vi "driveLoop.vi"() -> ()   [LabVIEW 2018]
uses:
  driveCommandEnum.ctl
  driveShifterEnum.ctl
  <vilib>/Platform/TimedLoop/XDataNode/timing_clust.ctl
  <vilib>/Platform/TimedLoop/XDataNode/nitl_modes.ctl
  <vilib>/Platform/TimedLoop/XDataNode/wakeup.ctl
  <userlib>/836-Library/System/TDMS_V2/Support/TDMS_DevRef.ctl
  <userlib>/836-Library/System/TDMS_V2/Support/Logging_Settings.ctl
  <userlib>/836-Library/System/TDMS_V2/Support/Group_FIFO_Config.ctl
  <userlib>/836-Library/System/TDMS_V2/Support/Channel_FIFO_Config.ctl
  driveStateEnum.ctl
  <vilib>/Rock Robotics/WPI/ThirdParty/Phoenix-LabVIEW/Motor Controller/Controls/CTRE_Phoenix_MotorControl_MotionProfileControlMode.ctl
  Climb/driveClimbStateEnum.ctl
  gear notifier.ctl
  <vilib>/Rock Robotics/WPI/ThirdParty/Phoenix-LabVIEW/Motor Controller/Controls/CTRE_Phoenix_MotorControl_ControlMode.ctl
  <vilib>/Rock Robotics/WPI/ThirdParty/Phoenix-LabVIEW/Motor Controller/Get/CTRE_Phoenix_MotorController_GetVoltage.vi
  <vilib>/addons/control/pid/pid.llb/PID (DBL).vi
  <vilib>/platform/TimedLoop/XDataNode/XDataNode.xnode
  <vilib>/Platform/TimedLoop/XDataNode/XDNodeRunTimeDep.lvlib
  <vilib>/addons/control/pid/NI_PID_pid.lvlib
panel:
  in  "LA limit throt wheel":dbl=0.6
  in  "LA limit throttle":dbl=1.0
  in  "aproachTargetSpeed":dbl=0.64
  in  "sonarBrakeAngleCone":dbl=20.0 format="%#_13g"
  in  "RocketSonarStandOff":dbl=11.0 format="%#_13g"
  in  "coast":dbl=0.08
  in  "alignAngleSetpoint":dbl(slide)=20.0 scale=-30.0..30.0
  in  "Enum":T1
  out "Power output":dbl(graph)=-0.1276953125
  out "Offset Angle":dbl(graph)=4.560546875
  in  "Turn High PID gains":T2={"proportional gain (Kc)"=0.039, "integral time (Ti, min)"=0.0, "derivative time (Td, min)"=0.0018000000000000004} {"derivative time (Td, min)" format="%.4f"; "integral time (Ti, min)" format="%.4f"; "proportional gain (Kc)" format="%.4f"}
  in  "Turn Low PID gains":T2={"proportional gain (Kc)"=0.027999999999999997, "integral time (Ti, min)"=0.0, "derivative time (Td, min)"=0.0018000000000000004} {"derivative time (Td, min)" format="%.4f"; "integral time (Ti, min)" format="%.4f"; "proportional gain (Kc)" format="%.4f"}
  in  "CutoutSonarStandOff":dbl=11.0 format="%#_13g"
  in  "Square?":bool=TRUE
  out "Iteration Duration":i64(graph)=2
  in  "Quickturn_Sens_Low":dbl=1.0
  in  "Quickturn_Sens_High":dbl=0.6 format="%#_13g"
  out "notification":T3=enum."Manuel"
  in  "limit":dbl=1.0
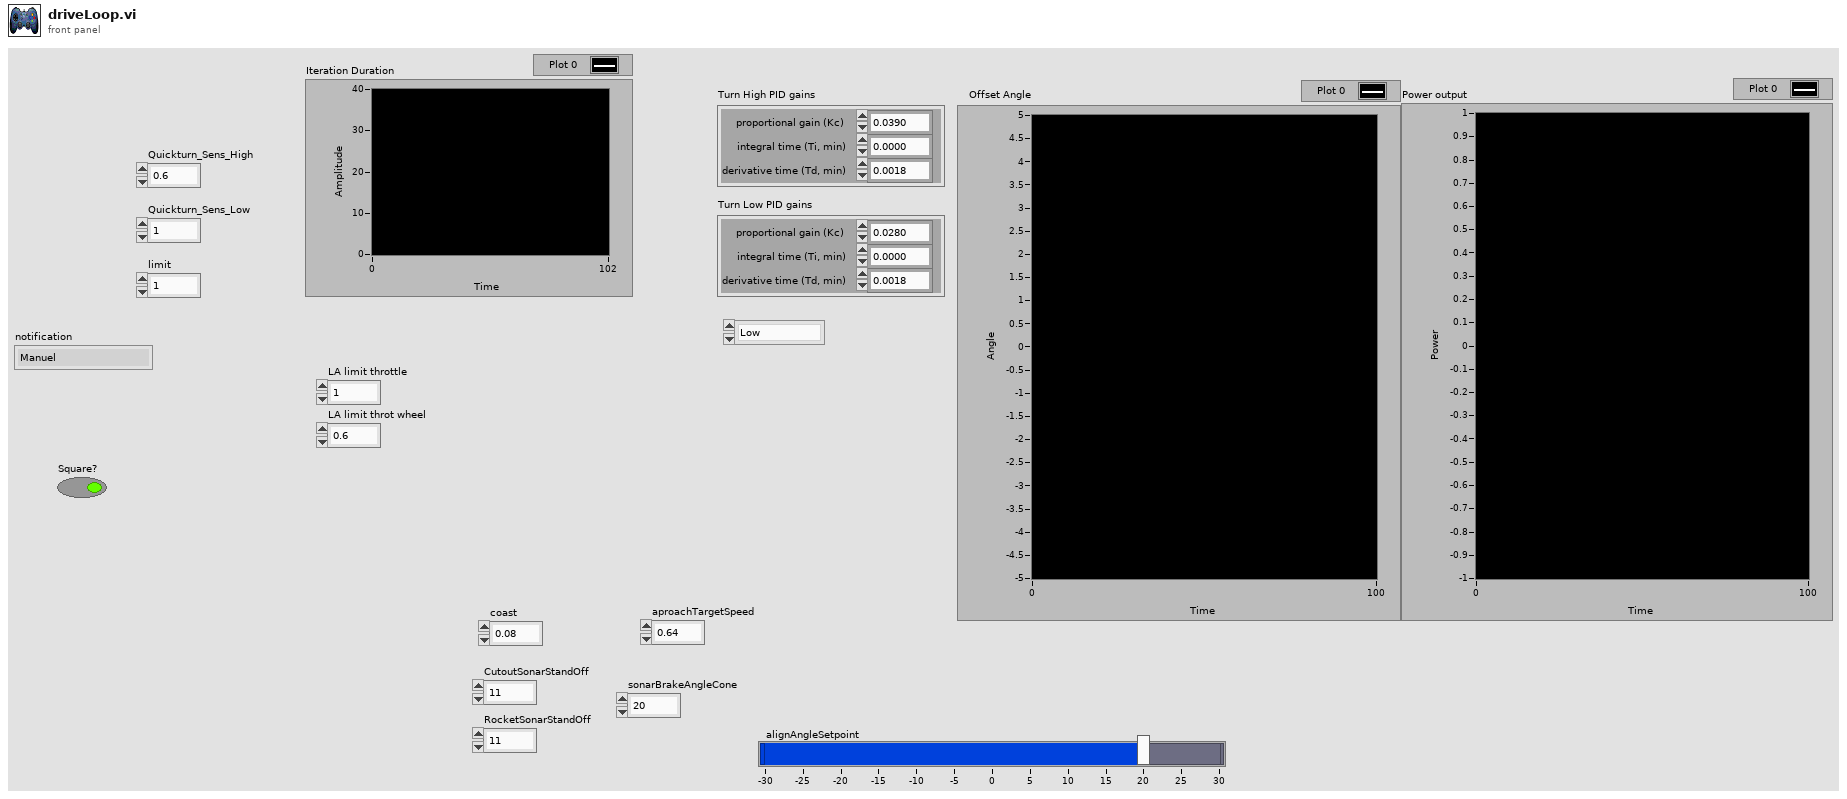
[diagram p1: front panel]
types:
  T1 = typedef "driveShifterEnum.ctl" = enum16{"Low", "High"}
  T2 = cluster{"proportional gain (Kc)":dbl, "integral time (Ti, min)":dbl, "derivative time (Td, min)":dbl}
  T3 = typedef "driveCommandEnum.ctl" = enum16{"doNothing", "Manuel", "Teleop", "Move to Target", "Climb", "Line Align", "Sonar BrakeTele", "Turn To Angle", "Auto Drive", "Test Auto Forward", "Test Auto Reversed", "Code Drive"}
  T4 = typedef "WPI_MotorControlDeviceRef.ctl" = cluster{"DeviceStatus":errorcluster, "Type":T5, "PWM":cluster{"PWM Channel":T6, "DeadBand":T7}, "CAN":cluster{"Device Number":u8, "SetOutput VI Ref":variant, "GetOutput VI Ref":variant, "Enable VI Ref":variant, "Disable VI Ref":variant, "Data":variant}, "Invert":bool, "DIO PWM":cluster{"PWM \"Enable\" Channel":T6, "DIOChannel":T8, "PWM Rate":dbl}}
  T5 = typedef "WPI_MotorControlType.ctl" = enum16{"PWM", "CAN", "DIO PWM"}
  T6 = typedef "FPGA_DIOPWMChannel.ctl" = enum8{"PWM 0", "PWM 1", "PWM 2", "PWM 3", "PWM 4", "PWM 5", "PWM 6", "PWM 7", "PWM 8", "PWM 9", "PWM MXP 0", "PWM MXP 1", "PWM MXP 2", "PWM MXP 3", "PWM MXP 4", "PWM MXP 5", "PWM MXP 6", "PWM MXP 7", "PWM MXP 8", "PWM MXP 9", "Invalid"}
  T7 = typedef "WPI_PWMDeadband.ctl" = cluster{"Name":string, "maxPositivePwm":i32, "minPositivePwm":i32, "centerPwm":i32, "maxNegativePwm":i32, "minNegativePwm":i32, "angularRange":u16}
  T8 = typedef "FPGA_DIOChannel.ctl" = enum8{"DIO 0", "DIO 1", "DIO 2", "DIO 3", "DIO 4", "DIO 5", "DIO 6", "DIO 7", "DIO 8", "DIO 9", "DIO MXP 0", "DIO MXP 1", "DIO MXP 2", "DIO MXP 3", "DIO MXP 4", "DIO MXP 5", "DIO MXP 6", "DIO MXP 7", "DIO MXP 8", "DIO MXP 9", "DIO MXP 10", "DIO MXP 11", "DIO MXP 12", "DIO MXP 13", "DIO MXP 14", "DIO MXP 15", "SPI Port CS1", "SPI Port CS2", "SPI Port CS3", "SPI Port MISO", "SPI Port MOSI", "Invalid"}
  T9 = typedef "CTRE_PigeonIMU_DeviceRef.ctl" = cluster{"DeviceStatus":errorcluster, "Device Number":u8, "Type":T10, "Device ID":u32, "Handle":u64, "UsageFrame":u32, "Library Path":path}
  T10 = typedef "CTRE_PigeonIMU_ConnectionType.ctl" = u32
  T11 = typedef "XDNodeRunTimeDep.lvlib/timing_clust.ctl" = cluster{"Expected End [f-1]":u64, "Actual End [f-1]":u64, "Finished Late? [f-1]":bool, "Expected End [i-1]":u64, "Actual End [i-1]":u64, "Finished Late? [i-1]":bool, "Expected Start [i]":u64, "Actual Start [i]":u64, "Expected Start [f]":u64, "Actual Start [f]":u64, "Source Name":string, "Structure Name":string, "Period":i64, "Deadline":i64, "Offset":i64, "Start":i64, "Priority":i32, "Timeout":i32, "Mode":T12, "Wakeup Reason":T13, "Error":errorcluster, "Source Type":string, "Secondary Source Type":string, "Global End Time":u64, "Global Start Time":u64, "Frame Duration":u64, "Iteration Duration":u64, "Assigned CPU":i32, "I/O Scan Engine Mode":u32}
  T12 = typedef "XDNodeRunTimeDep.lvlib/nitl_modes.ctl" = enum32{"No Change", "Process missed periods, maintain original phase", "Discard missed periods, maintain original phase", "Process missed periods, ignore original phase", "Discard missed periods, ignore original phase"}
  T13 = typedef "XDNodeRunTimeDep.lvlib/wakeup.ctl" = enum32{"Normal", "Aborted", "Asynchronous wakeup", "Timing source error", "Timed loop error", "Timeout"}
  T14 = typedef "driveStateEnum.ctl" = enum16{"doNothing", "Manuel", "Teleop", "Follow Path (init)", "Follow Path", "Move to Target", "Climb", "Line Align", "Turn to Angle", "Sonar Brake Tele", "Code Drive"}
  T15 = enum16{"FollowerType_PercentOutput", "FollowerType_AuxOutput1"}
  T16 = cluster{"Quickturn_Sens_High":dbl, "Quickturn_Sens_Low":dbl}
  T17 = typedef "CTRE_Phoenix_MotorControl_MotionProfileControlMode.ctl" = u16
  T18 = typedef "CTRE_Phoenix_MotorControl_BufferedTrajectoryPointStream_DeviceRef.ctl" = cluster{"Handle":u64, "Library Path":path}
  T19 = typedef "driveClimbStateEnum.ctl" = enum16{"Do Nothing", "Drive Forward"}
  T20 = typedef "gear notifier.ctl" = cluster{"High Gear?":bool, "Low Gear?":bool}
  T21 = typedef "CTRE_Phoenix_MotorControl_ControlMode.ctl" = u16
  T22 = typedef "TDMS_DevRef.ctl" = cluster{"Name":string, "File Ref":refnum<k34>, "Start Time":timestamp, "Logging Settings":T23, "Group FIFO Config":T24[], "Data To Write":refnum<data-value>, "semaphore":T26, "Ref Time Reset":refnum<k4>}
  T23 = typedef "Logging_Settings.ctl" = cluster{"Data Grab Period":dbl, "File Write Period":dbl, "Max Stored Size":dbl, "Burst Size":dbl}
  T24 = typedef "Group_FIFO_Config.ctl" = cluster{"Group":string, "Channels":T25[], "Channel Names":string[]}
  T25 = typedef "Channel_FIFO_Config.ctl" = cluster{"Channel":string, "FIFO":refnum<k33>}
  T26 = typedef "Semaphore RefNum" = refnum<k1>
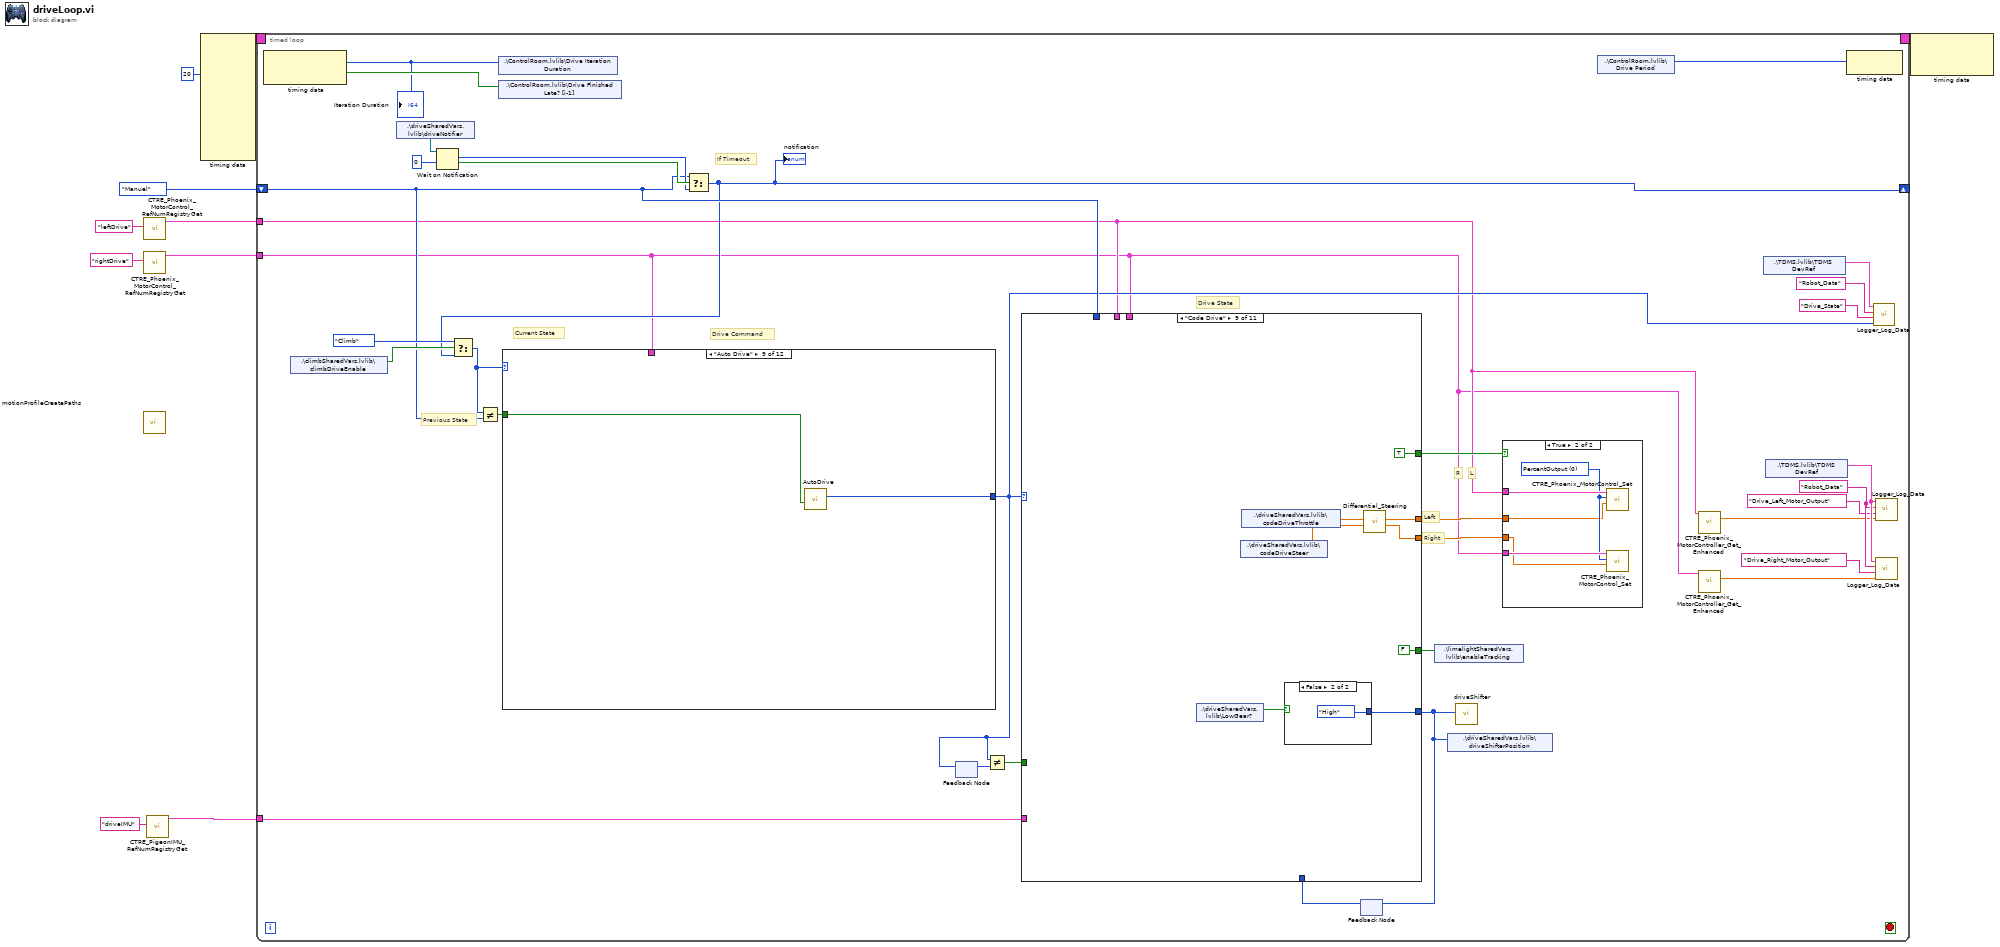
[diagram p0: block diagram]
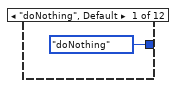
[diagram p2: hidden frame]
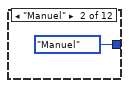
[diagram p3: hidden frame]
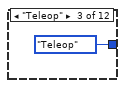
[diagram p4: hidden frame]
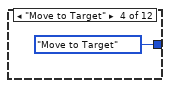
[diagram p5: hidden frame]
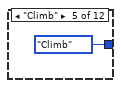
[diagram p6: hidden frame]
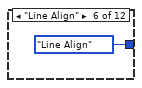
[diagram p7: hidden frame]
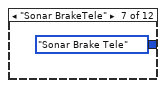
[diagram p8: hidden frame]
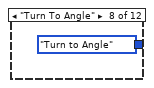
[diagram p9: hidden frame]
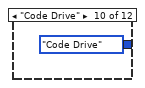
[diagram p10: hidden frame]
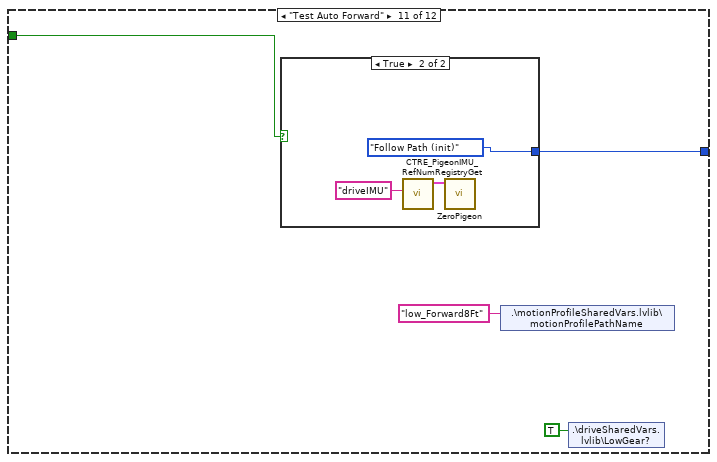
[diagram p11: hidden frame]
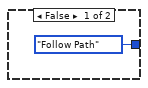
[diagram p12: hidden frame]
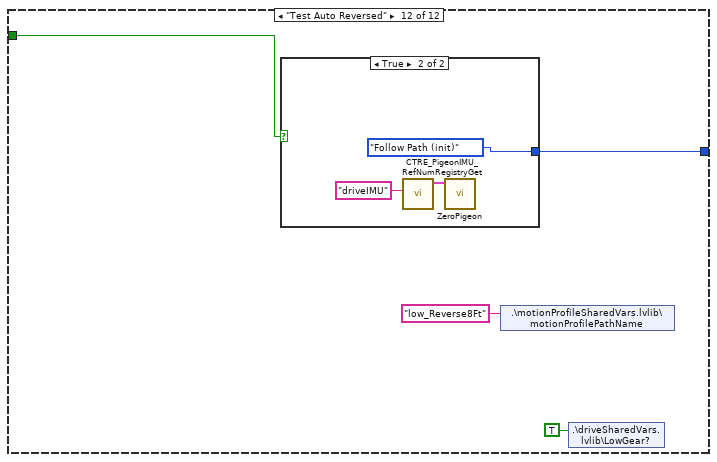
[diagram p13: hidden frame]
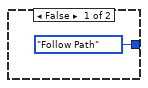
[diagram p14: hidden frame]
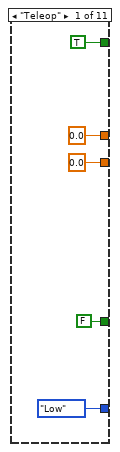
[diagram p16: hidden frame]
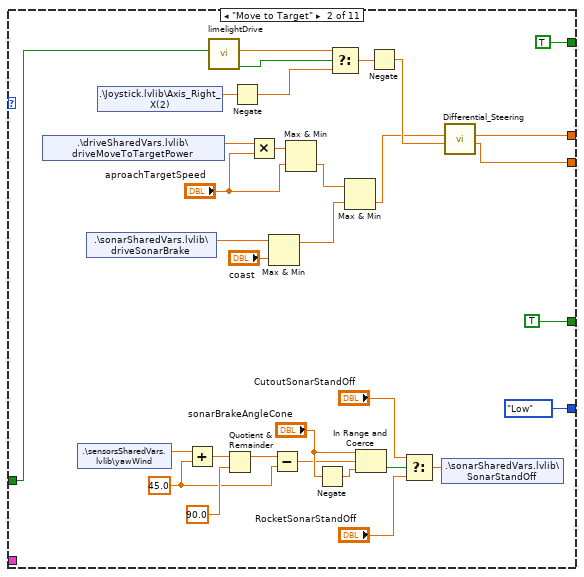
[diagram p17: hidden frame]
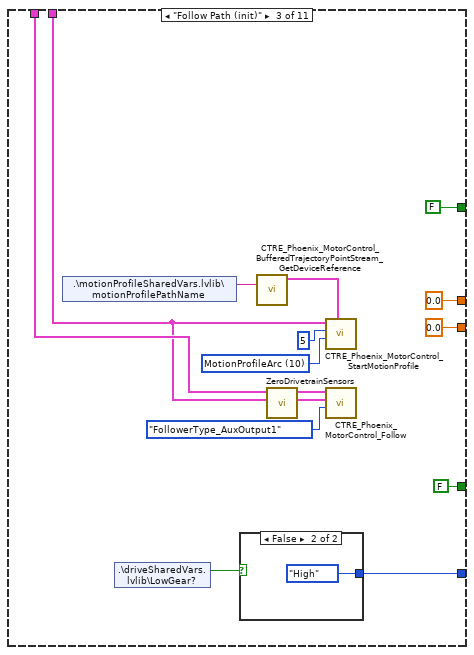
[diagram p18: hidden frame]
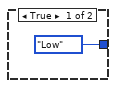
[diagram p19: hidden frame]
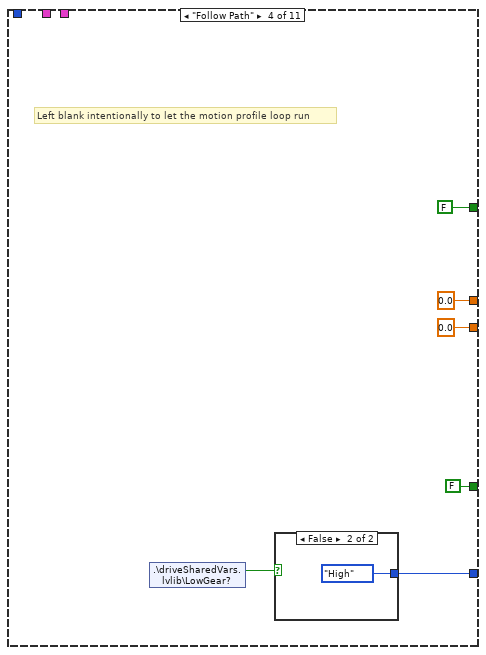
[diagram p20: hidden frame]
diagram:
  n1 = call "motionProfileCreatePaths.vi"() -> ()  [unwired: 12 in]
  n2 = call <vilib>:"CTRE_Phoenix_MotorControl_RefNumRegistryGet.vi"("refnum name"="leftDrive") -> ("PhoenixMotorControlDevRef"=w5:T4)  [unwired: 9 in, 1 out]
  n3 = call <vilib>:"CTRE_Phoenix_MotorControl_RefNumRegistryGet.vi"("refnum name"="rightDrive") -> ("PhoenixMotorControlDevRef"=w4:T4)  [unwired: 9 in, 1 out]
  n4 = call <vilib>:"CTRE_PigeonIMU_RefNumRegistryGet.vi"("refnum name"="driveIMU") -> ("PigeonIMUDevRef"=w2:T9)  [unwired: 9 in, 1 out]
  n5 = node-c288(20 ("Priority")) -> (w10:T11)  [unwired: 9 in]
  n6 = timed-loop {
    timing: w10 -> [_]
    timing-out: [_] -> w9
    shift-right: [w28] -> _
    shift-left: driveCommandEnum."Manuel" ("Drive State Enum") -> [w29]
    tunnel: w5 -> [w12]
    tunnel: w4 -> [w11]
    tunnel: w2 -> [w41]
    stop <- _ stop-if-true
    w22 = "Robot_Data" ("Group")
    # "Drive Command"
    # "Drive State"
    # "Previous State"
    # "Current State"
    # "Right"
    # "Left"
    # "L"
    # "R"
    # "If Timeout"
    n7 = node-c288() -> (w30:i64, w31:bool)  [unwired: 1 in]
    "Iteration Duration" <- w30
    n8 = shared-variable ".\\climbSharedVars.lvlib\\climbDriveEnable"() -> (w36:bool)  [unwired: 1 in, 1 out]
    n9 = shared-variable ".\\driveSharedVars.lvlib\\driveNotifier"() -> (w25:refnum<notifier>)  [unwired: 1 in, 1 out]
    n10 = Wait on Notification(notifier=w25, timeout in ms (-1)=0) -> (notification=w33:T3, timed out?=w44:bool)  [unwired: 2 in, 2 out]
    n11 = shared-variable ".\\ControlRoom.lvlib\\Drive Iteration Duration"(w30) -> ()  [unwired: 1 in, 1 out]
    n12 = shared-variable ".\\ControlRoom.lvlib\\Drive Finished Late? [i-1]"(w31) -> ()  [unwired: 1 in, 1 out]
    n13 = Select(t=w29, s=w44, f=w33) -> (s? t:f=w28:T3)
    "notification" <- w28
    n14 = Select(t=driveCommandEnum."Climb" ("f"), s=w36, f=w28) -> (s? t:f=w38:T3)
    n15 = Not Equal?(x=w38, y=w29) -> (x != y?=w39:bool)
    n16 = case shown="\"Auto Drive\"" w38 {
      tunnel: w39 -> [_ _ _ _ _ _ _ _ w53 _ w59 w67]
      tunnel: [driveStateEnum."doNothing" ("Drive State Enum") driveStateEnum."Manuel" ("Drive State Enum") driveStateEnum."Teleop" ("Drive State Enum") driveStateEnum."Move to Target" ("Drive State Enum") driveStateEnum."Climb" ("Drive State Enum") driveStateEnum."Line Align" ("Drive State Enum") driveStateEnum."Sonar Brake Tele" ("Drive State Enum") driveStateEnum."Turn to Angle" ("Drive State Enum") w54 driveStateEnum."Code Drive" ("Drive State Enum") w58 w66] -> w15
      tunnel: w11 -> [_ _ _ _ _ _ _ _ _ _ _ _]
      frame "doNothing", Default {
      }
      frame "Manuel" {
      }
      frame "Teleop" {
      }
      frame "Move to Target" {
      }
      frame "Climb" {
      }
      frame "Line Align" {
      }
      frame "Sonar BrakeTele" {
      }
      frame "Turn To Angle" {
      }
      frame "Auto Drive" {
        n17 = call "AutoDrive.vi"("Initialized"=w53) -> ("Drive State"=w54:T14)  [unwired: 10 in]
      }
      frame "Code Drive" {
      }
      frame "Test Auto Forward" {
        n18 = case shown="True" w59 {
          tunnel: [driveStateEnum."Follow Path" ("Drive State") driveStateEnum."Follow Path (init)" ("Drive State")] -> w58
          frame False {
          }
          frame True {
            n19 = call <vilib>:"CTRE_PigeonIMU_RefNumRegistryGet.vi"("refnum name"="driveIMU") -> ("PigeonIMUDevRef"=w61:T9)  [unwired: 9 in, 1 out]
            n20 = call "ZeroPigeon.vi"("Pigeon"=w61) -> ()  [unwired: 8 in, 1 out]
          }
        }
        n21 = shared-variable ".\\motionProfileSharedVars.lvlib\\motionProfilePathName"("low_Forward8Ft" ("motionProfilePathName")) -> ()  [unwired: 1 in, 1 out]
        n22 = shared-variable ".\\driveSharedVars.lvlib\\LowGear?"(TRUE ("LowGear?")) -> ()  [unwired: 1 in, 1 out]
      }
      frame "Test Auto Reversed" {
        n23 = case shown="True" w67 {
          tunnel: [driveStateEnum."Follow Path" ("Drive State") driveStateEnum."Follow Path (init)" ("Drive State")] -> w66
          frame False {
          }
          frame True {
            n24 = call <vilib>:"CTRE_PigeonIMU_RefNumRegistryGet.vi"("refnum name"="driveIMU") -> ("PigeonIMUDevRef"=w69:T9)  [unwired: 9 in, 1 out]
            n25 = call "ZeroPigeon.vi"("Pigeon"=w69) -> ()  [unwired: 8 in, 1 out]
          }
        }
        n26 = shared-variable ".\\motionProfileSharedVars.lvlib\\motionProfilePathName"("low_Reverse8Ft" ("motionProfilePathName")) -> ()  [unwired: 1 in, 1 out]
        n27 = shared-variable ".\\driveSharedVars.lvlib\\LowGear?"(TRUE ("LowGear?")) -> ()  [unwired: 1 in, 1 out]
      }
    }
    n28 = feedback-in #1(w15) -> ()
    n29 = feedback #1() -> (w17:T14)  [unwired: 1 in]
    n30 = Not Equal?(x=w15, y=w17) -> (x != y?=w16:bool)
    n31 = feedback #2() -> (w34:T1)  [unwired: 1 in]
    n32 = case shown="\"Code Drive\"" w15 {
      tunnel: [0.0 ("Throttle") w103 0.0 ("Throttle") 0.0 ("Throttle") w141 w156 0.0 ("Throttle") w198 w209 w218 w228] -> w43
      tunnel: [0.0 ("Wheel") w102 0.0 ("Wheel") 0.0 ("Wheel") w141 w155 0.0 ("Wheel") w197 w210 w219 w227] -> w42
      tunnel: w41 -> [_ _ _ _ _ _ _ _ _ _ _]
      tunnel: w12 -> [_ _ w126 _ _ _ _ _ _ _ _]
      tunnel: w11 -> [_ _ w125 _ _ _ _ _ _ _ _]
      tunnel: w29 -> [_ _ _ _ _ _ _ _ _ _ _]
      tunnel: [TRUE ("x .and. y?") TRUE ("x .and. y?") FALSE ("x .and. y?") FALSE ("x .and. y?") TRUE ("x .and. y?") TRUE ("x .and. y?") TRUE ("x .and. y?") TRUE ("x .and. y?") TRUE ("x .and. y?") TRUE ("x .and. y?") TRUE ("x .and. y?")] -> w40
      tunnel: [driveShifterEnum."Low" driveShifterEnum."Low" w114 w131 w143 driveShifterEnum."High" driveShifterEnum."High" w191 w206 driveShifterEnum."Low" ("Enum") "Enum"] -> w35
      tunnel: w34 -> [_ _ _ _ w143 _ _ _ _ _ _]
      tunnel: [FALSE TRUE FALSE FALSE FALSE FALSE FALSE FALSE FALSE FALSE FALSE] -> w27
      tunnel: w16 -> [_ w82 _ _ _ _ _ _ _ w215 _]
      frame "Teleop" {
      }
      frame "Move to Target" {
        w87 = 45.0 ("y")
        n33 = shared-variable ".\\driveSharedVars.lvlib\\driveMoveToTargetPower"() -> (w86:dbl)  [unwired: 1 in, 1 out]
        n34 = shared-variable ".\\sensorsSharedVars.lvlib\\yawWind"() -> (w98:dbl)  [unwired: 1 in, 1 out]
        n35 = shared-variable ".\\sonarSharedVars.lvlib\\driveSonarBrake"() -> (w101:dbl)  [unwired: 1 in, 1 out]
        n36 = shared-variable ".\\Joystick.lvlib\\Axis_Right_X(2)"() -> (w109:dbl)  [unwired: 1 in, 1 out]
        n37 = Add(x=w98, y=w87) -> (x+y=w89:dbl)
        n38 = call "limelightDrive.vi"("reinitialize? (F)"=w82) -> ("Valid Track"=w110:bool, "Turn Output"=w111:dbl)  [unwired: 9 in]
        n39 = Quotient & Remainder(x=w89, y=90.0) -> (x-y*floor(x/y)=w96:dbl)  [unwired: 1 out]
        n40 = Negate(x=w109) -> (-x=w108:dbl)
        n41 = Multiply(x=w86, y="aproachTargetSpeed") -> (x*y=w85:dbl)
        n42 = Max & Min(x=w101, y="coast") -> (max(x,y)=w99:dbl)  [unwired: 1 out]
        n43 = Subtract(x=w96, y=w87) -> (x-y=w88:dbl)
        n44 = Max & Min(x=w85, y="aproachTargetSpeed") -> (min(x,y)=w83:dbl)  [unwired: 1 out]
        n45 = Negate(x="sonarBrakeAngleCone") -> (-x=w94:dbl)
        n46 = Select(t=w111, s=w110, f=w108) -> (s? t:f=w106:dbl)
        n47 = Max & Min(x=w83, y=w99) -> (min(x,y)=w104:dbl)  [unwired: 1 out]
        n48 = In Range and Coerce(upper limit="sonarBrakeAngleCone", x=w88, lower limit=w94) -> (In Range?=w93:bool)  [unwired: 1 out]
        n49 = Negate(x=w106) -> (-x=w105:dbl)
        n50 = Select(t="CutoutSonarStandOff", s=w93, f="RocketSonarStandOff") -> (s? t:f=w92:dbl)
        n51 = shared-variable ".\\sonarSharedVars.lvlib\\SonarStandOff"(w92) -> ()  [unwired: 1 in, 1 out]
        n52 = call <userlib>:"Differential_Steering.vi"("Steer"=w105, "Base"=w104) -> ("Right"=w102:dbl, "Left"=w103:dbl)  [unwired: 4 in]
      }
      frame "Follow Path (init)" {
        w121 = T17 10 items=["MotionProfile"=6, "MotionProfileArc"=10] ("Control Mode")
        n53 = shared-variable ".\\motionProfileSharedVars.lvlib\\motionProfilePathName"() -> (w117:string)  [unwired: 1 in, 1 out]
        n54 = shared-variable ".\\driveSharedVars.lvlib\\LowGear?"() -> (w115:bool)  [unwired: 1 in, 1 out]
        n55 = case shown="False" w115 {
          tunnel: [driveShifterEnum."Low" ("Enum") driveShifterEnum."High" ("Enum")] -> w114
          frame True {
          }
          frame False {
          }
        }
        n56 = call <vilib>:"CTRE_Phoenix_MotorControl_BufferedTrajectoryPointStream_GetDeviceReference.vi"("refnum name"=w117) -> ("BufferedTrajectoryPointStream_DevRef"=w118:T18)  [unwired: 9 in, 1 out]
        n57 = call "ZeroDrivetrainSensors.vi"("Talon 2"=w125, "Talon 1"=w126) -> ("Talon 2"=w119:T4, "Talon 1"=w120:T4)  [unwired: 8 in]
        n58 = call <vilib>:"CTRE_Phoenix_MotorControl_StartMotionProfile.vi"("BufferedTrajectoryPointStream_DevRef"=w118, "Control Mode"=w121, "minBufferedPts"=u32 5, "PhoenixMotorControlDevRef"=w125) -> ()  [unwired: 6 in, 2 out]
        n59 = call <vilib>:"CTRE_Phoenix_MotorControl_Follow.vi"("FollowerType"=T15."FollowerType_AuxOutput1", "Master Controller to Follow"=w119, "PhoenixMotorControlDevRef"=w120) -> ()  [unwired: 7 in, 2 out]
      }
      frame "Follow Path" {
        # "Left blank intentionally to let the motion profile loop run"
        n60 = shared-variable ".\\driveSharedVars.lvlib\\LowGear?"() -> (w132:bool)  [unwired: 1 in, 1 out]
        n61 = case shown="False" w132 {
          tunnel: [driveShifterEnum."Low" ("Enum") driveShifterEnum."High" ("Enum")] -> w131
          frame True {
          }
          frame False {
          }
        }
      }
      frame "Sonar Brake Tele" {
        # "Share Control Authority between\nDriver input and Sonar PID"
        n62 = shared-variable ".\\Joystick.lvlib\\Axis_Left_Y(1)"() -> (w140:dbl)  [unwired: 1 in, 1 out]
        n63 = shared-variable ".\\sonarSharedVars.lvlib\\driveSonarBrake"() -> (w142:dbl)  [unwired: 1 in, 1 out]
        n64 = Negate(x=w140) -> (-x=w139:dbl)
        n65 = Max & Min(x=w139, y=w142) -> (min(x,y)=w141:dbl)  [unwired: 1 out]
      }
      frame "Climb" {
        n66 = shared-variable ".\\driveSharedVars.lvlib\\driveClimbStateNotifier"() -> (w152:refnum<notifier>)  [unwired: 1 in, 1 out]
        n67 = Wait on Notification(notifier=w152, timeout in ms (-1)=0) -> (notification=w148:T19, timed out?=w150:bool)  [unwired: 2 in, 2 out]
        n68 = feedback-in #3(w148) -> ()
        n69 = feedback #3() -> (w147:T19)  [unwired: 1 in]
        n70 = Select(t=w147, s=w150, f=w148) -> (s? t:f=w149:T19)
        n71 = case shown="\"Drive Forward\"" w149 {
          tunnel: [w157 w159] -> w156
          tunnel: [w157 w158] -> w155
          frame "Drive Forward" {
            n72 = shared-variable ".\\climbSharedVars.lvlib\\Drive Speed"() -> (w157:dbl)  [unwired: 1 in, 1 out]
          }
          frame "Do Nothing", Default {
            w158 = 0.0  # Right
            w159 = 0.0  # Left
          }
        }
      }
      frame "doNothing", Default {
      }
      frame "Manuel" {
        n73 = shared-variable ".\\driveSharedVars.lvlib\\driveShifterNotifier"() -> (w165:refnum<notifier>)  [unwired: 1 in, 1 out]
        n74 = shared-variable ".\\Joystick.lvlib\\Axis_Right_X(2)"() -> (w168:dbl)  [unwired: 1 in, 1 out]
        n75 = shared-variable ".\\Joystick.lvlib\\Axis_Left_Y(1)"() -> (w172:dbl)  [unwired: 1 in, 1 out]
        n76 = Wait on Notification(notifier=w165, timeout in ms (-1)=0) -> (notification=w180:T20, timed out?=w179:bool)  [unwired: 2 in, 2 out]
        n77 = Sign(1:w172) -> (0:w176:dbl)
        n78 = Sign(1:w168) -> (0:w174:dbl)
        n79 = Square(x=w172) -> (x^2=w177:dbl)
        n80 = Square(x=w168) -> (x^2=w175:dbl)
        n81 = feedback #4() -> (w178:T20)  [unwired: 1 in]
        n82 = Select(t=w178, s=w179, f=w180) -> (s? t:f=w182:T20)
        n83 = feedback-in #4(w182) -> ()
        n84 = Bundle By Name(cluster=T16 {"Quickturn_Sens_High"=1.0, "Quickturn_Sens_Low"=1.0} ("Sens Values"), "Quickturn_Sens_High"="Quickturn_Sens_High", "Quickturn_Sens_Low"="Quickturn_Sens_Low") -> (w194:T16)
        n85 = Multiply(x=w177, y=w176) -> (x*y=w173:dbl)
        n86 = Multiply(x=w175, y=w174) -> (x*y=w170:dbl)
        n87 = Select(t=w173, s="Square?", f=w172) -> (s? t:f=w171:dbl)
        n88 = Select(t=w170, s="Square?", f=w168) -> (s? t:f=w169:dbl)
        n89 = Unbundle By Name(w182) -> ("High Gear?"=w183:bool, "Low Gear?"=w184:bool)
        n90 = Negate(x=w171) -> (-x=w202:dbl)
        n91 = Multiply(x=w202, y="limit") -> (x*y=w166:dbl)
        n92 = Multiply(x="limit", y=w169) -> (x*y=w199:dbl)
        n93 = call <userlib>:"JK_Latch.vi"("Reset"=w183, "Set"=w184) -> ("Q"=w185:bool)  [unwired: 5 in]
        n94 = Select(t=driveShifterEnum."Low", s=w185, f=driveShifterEnum."High") -> (s? t:f=w191:T1)
        n95 = case shown="\"Low\"" w191 {
          tunnel: [enum16{"low", "high"}."high" ("gear shift state") enum16{"low", "high"}."low" ("gear shift state")] -> w190
          frame "High" {
          }
          frame "Low" {
          }
        }
        n96 = call <userlib>:"hmi_cheesy_drive.vi"("Sens Values"=w194, "gear shift state"=w190, "Quick Turn"=TRUE, "Wheel"=w199, "Throttle"=w166) -> ("Drive Data"=w201:cluster{"Left":dbl, "Right":dbl})  [unwired: 6 in]
        n97 = Unbundle By Name(w201) -> ("Left"=w198:dbl, "Right"=w197:dbl)
      }
      frame "Code Drive" {
        n98 = shared-variable ".\\driveSharedVars.lvlib\\LowGear?"() -> (w205:bool)  [unwired: 1 in, 1 out]
        n99 = shared-variable ".\\driveSharedVars.lvlib\\codeDriveSteer"() -> (w207:dbl)  [unwired: 1 in, 1 out]
        n100 = shared-variable ".\\driveSharedVars.lvlib\\codeDriveThrottle"() -> (w208:dbl)  [unwired: 1 in, 1 out]
        n101 = case shown="False" w205 {
          tunnel: [driveShifterEnum."Low" ("Enum") driveShifterEnum."High" ("Enum")] -> w206
          frame True {
          }
          frame False {
          }
        }
        n102 = call <userlib>:"Differential_Steering.vi"("Steer"=w207, "Base"=w208) -> ("Right"=w210:dbl, "Left"=w209:dbl)  [unwired: 4 in]
      }
      frame "Line Align" {
        n103 = call "Line Align&Snap 90.vi"("Init"=w215, "LA limit throt wheel"="LA limit throt wheel", "LA limit throttle"="LA limit throttle") -> ("Right"=w219:dbl, "Left"=w218:dbl)  [unwired: 7 in]
      }
      frame "Turn to Angle" {
        w233 = TRUE  # Invert Direction
        w234 = 10.0  # Trigger Range
        n104 = shared-variable ".\\sensorsSharedVars.lvlib\\driveIMUYawPitchRoll"() -> (w231:cluster{"Yaw":dbl, "Pitch":dbl, "Roll":dbl})  [unwired: 1 in, 1 out]
        n105 = shared-variable ".\\driveSharedVars.lvlib\\alignAngleSetpoint"() -> (w232:dbl)  [unwired: 1 in, 1 out]
        n106 = case shown="\"High\"" "Enum" {
          tunnel: ["Turn Low PID gains" "Turn High PID gains"] -> w238
          frame "Low", Default {
          }
          frame "High" {
          }
        }
        n107 = Negate(x=w232) -> (-x=w224:dbl)
        n108 = Unbundle By Name(w231) -> ("Yaw"=w237:dbl)
        n109 = shared-variable ".\\driveSharedVars.lvlib\\alignAngleSetpoint"("alignAngleSetpoint") -> ()  [unwired: 1 in, 1 out]
        n110 = call "TurnToAngle.vi"("Invert Direction"=w233, "Trigger Range"=w234, "Turn To"=w224, "Gyro"=w237) -> ("Triggered"=w229:bool, "Offset Angle"=w235:dbl)  [unwired: 6 in]
        "Offset Angle" <- w235
        n111 = shared-variable ".\\driveSharedVars.lvlib\\alignAngleTriggered"(w229) -> ()  [unwired: 1 in, 1 out]
        n112 = call-poly <vilib>:"PID.vi"("output range"=cluster{"output high":dbl, "output low":dbl} {"output high"=1.0, "output low"=-1.0}, "PID gains"=w238, "process variable"=w235, "setpoint"=0.0) -> ("output"=w226:dbl)  [unwired: 6 in, 1 out]
        "Power output" <- w226
        n113 = call <userlib>:"Differential_Steering.vi"("Steer"=w226, "Base"=0.0 ("Y axis value")) -> ("Right"=w227:dbl, "Left"=w228:dbl)  [unwired: 4 in]
      }
    }
    n114 = feedback-in #2(w35) -> ()
    n115 = shared-variable ".\\limelightSharedVars.lvlib\\enableTracking"(w27) -> ()  [unwired: 1 in, 1 out]
    n116 = shared-variable ".\\driveSharedVars.lvlib\\driveShifterPosition"(w35) -> ()  [unwired: 1 in, 1 out]
    n117 = call "driveShifter.vi"(10:w35) -> ()  [unwired: 11 in]
    n118 = case shown="True" w40 {
      tunnel: w12 -> [_ w76]
      tunnel: w11 -> [_ w75]
      tunnel: w43 -> [_ w72]
      tunnel: w42 -> [_ w73]
      frame False {
        # "Left Blank\nIntentionally\nfor Motion Profiling"
      }
      frame True {
        w74 = T21 0 items=["PercentOutput"=0, "Position"=1, "Velocity"=2, "Current"=3, "Follower"=5, "MotionProfile"=6, "MotionMagic"=7, "MotionProfileArc"=10, "Disabled"=15] ("Control Mode")
        n119 = call <vilib>:"CTRE_Phoenix_MotorControl_Set.vi"("Output"=w72, "Control Mode"=w74, "PhoenixMotorControlDevRef"=w76) -> ()  [unwired: 7 in, 2 out]
        n120 = call <vilib>:"CTRE_Phoenix_MotorControl_Set.vi"("Output"=w73, "Control Mode"=w74, "PhoenixMotorControlDevRef"=w75) -> ()  [unwired: 7 in, 2 out]
      }
    }
    n121 = shared-variable ".\\ControlRoom.lvlib\\Drive Period"() -> (w32:i64)  [unwired: 1 in, 1 out]
    n122 = call-poly <vilib>:"CTRE_Phoenix_MotorController_Get_Enhanced.vi"("PhoenixMotorControlDevRef"=w12) -> ("Percent Output"=w14:dbl)  [unwired: 10 in, 4 out]
    n123 = call-poly <vilib>:"CTRE_Phoenix_MotorController_Get_Enhanced.vi"("PhoenixMotorControlDevRef"=w11) -> ("Percent Output"=w13:dbl)  [unwired: 10 in, 4 out]
    n124 = shared-variable ".\\TDMS.lvlib\\TDMS DevRef"() -> (w19:T22)  [unwired: 1 in, 1 out]
    n125 = shared-variable ".\\TDMS.lvlib\\TDMS DevRef"() -> (w23:T22)  [unwired: 1 in, 1 out]
    n126 = node-c288(w32) -> ()  [unwired: 1 out]
    n127 = call <userlib>:"Logger_Log_Data.vi"("Data"=w15, "Channel"="Drive_State", "Group"="Robot_Data", "TDMS DevRef"=w19) -> ()  [unwired: 7 in, 1 out]
    n128 = call <userlib>:"Logger_Log_Data.vi"("Data"=w14, "Channel"="Drive_Left_Motor_Output", "Group"=w22, "TDMS DevRef"=w23) -> ()  [unwired: 7 in, 1 out]
    n129 = call <userlib>:"Logger_Log_Data.vi"("Data"=w13, "Channel"="Drive_Right_Motor_Output", "Group"=w22, "TDMS DevRef"=w23) -> ()  [unwired: 7 in, 1 out]
  }
  n130 = node-c288(w9) -> ()  [unwired: 2 out]
